vi "Get RemIO Write Scaling Factor.vi"(8 "error in (no error)":errorcluster, 10 "RemIO Module in":refnum<class "RemIO Module.lvclass">, 11 "Node Ptr In":T1 format="%.0x") -> (0 "error out":errorcluster, 1 "Scaling Factors":dbl[](array[numeric]), 2 "RemIO Module out":refnum<class "RemIO Module.lvclass">, 3 "Node Ptr Out":T1 format="%.0x", 5 "Per Channel?":bool)   [LabVIEW 2016, in "Modules.lvlib" / "RemIO Module.lvclass"]
doc: "This VI Returns the scaling factors for REM IO Output Modules"
uses:
  RemIO Module.lvclass
  <vilib>/NI Veristand/Custom Device API/Custom Device Item Ref.ctl
  <vilib>/NI Veristand/Custom Device API/Custom Device API.lvlib
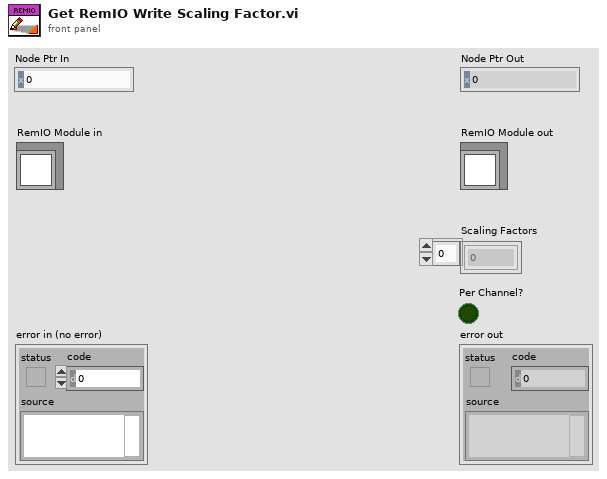
[diagram p1: front panel]
types:
  T1 = typedef "Custom Device API.lvlib/Custom Device Item Ref.ctl" = u64
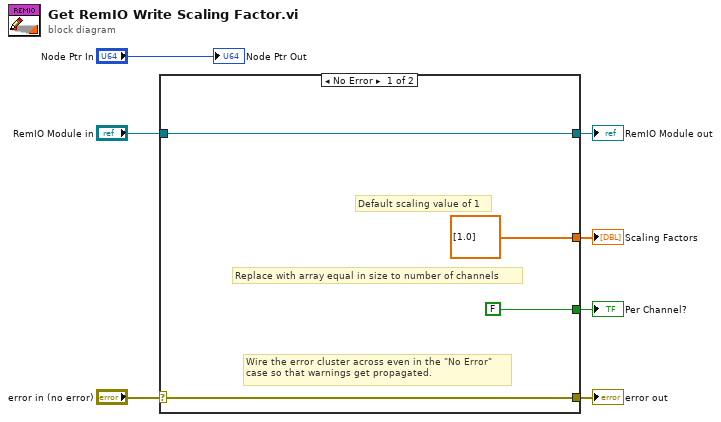
[diagram p0: block diagram]
diagram:
  n1 = case shown="No Error" "error in (no error)" {
    selector: "error in (no error)" -> [w10 w13]
    tunnel: [w10 w13] -> w6
    tunnel: [w11 w12] -> w4
    tunnel: "RemIO Module in" -> [w11 w12]
    tunnel: [dbl[] [1.0] _] -> w3
    tunnel: [FALSE _] -> w1
    frame No Error {
      # "Replace with array equal in size to number of channels"
      # "Default scaling value of 1"
      # "Wire the error cluster across even in the \"No Error\"\ncase so that warnings get propagated."
    }
    frame Error {
    }
  }
  "error out" <- w6
  "RemIO Module out" <- w4
  "Scaling Factors" <- w3
  "Per Channel?" <- w1
  "Node Ptr Out" <- "Node Ptr In"
